vi "Untitled 2.vi"() -> ()   [LabVIEW 2020]
uses:
  <vilib>/Utility/NIReport.llb/NI_report.lvclass
  <vilib>/addons/_office/NI_ReportGenerationToolkit.lvlib
panel:
  out "String":string
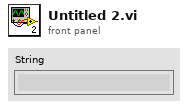
[diagram p1: front panel]
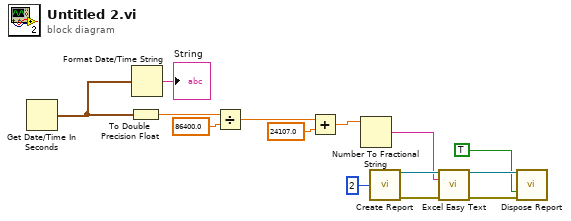
[diagram p0: block diagram]
diagram:
  n1 = Get Date/Time In Seconds() -> (seconds since 1Jan1904=w7:timestamp)
  n2 = To Double Precision Float(number=w7) -> (double precision float=w4:dbl)
  n3 = Format Date/Time String(seconds (now)=w7) -> (date/time string=→"String":string)  [unwired: 2 in]
  n4 = Divide(x=w4, y=86400.0) -> (x/y=w2:dbl)
  n5 = Add(x=w2, y=24107.0) -> (x+y=w1:dbl)
  n6 = Number To Fractional String(number=w1) -> (F-format string=w6:string)  [unwired: 3 in]
  n7 = call <vilib>:"Create Report.vi"("report type"=2) -> ("report out"=w12:refnum<class "NI_report.lvclass">, "error out"=w13:errorcluster)  [unwired: 13 in]
  n8 = call <vilib>:"Excel Easy Text.vi"("report in"=w12, "text"=w6, "error in (no error)"=w13) -> ("report out"=w9:refnum<class "NI_report.lvclass">, "error out"=w10:errorcluster)  [unwired: 8 in, 3 out]
  n9 = call-dynamic "Dispose Report.vi"("report in"=w9, "save changes? (F)"=TRUE, "error in (no error)"=w10) -> ()  [unwired: 12 in, 1 out]
